vi "matrix-transpose-encapsulate.vi"(11 "output matrix in":T1) -> (3 "output matrix out":T1)   [LabVIEW 2019]
uses:
  <vilib>/Analysis/Matrix/Datatypes/RealMatrix.ctl
  <vilib>/Analysis/Matrix/NI_Matrix.lvlib
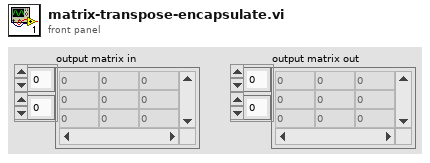
[diagram p1: front panel]
types:
  T1 = typedef "NI_Matrix.lvlib/RealMatrix.ctl" = dbl[][]
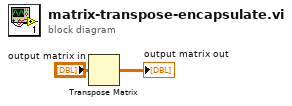
[diagram p0: block diagram]
diagram:
  n1 = Transpose Matrix(1:"output matrix in") -> (0:→"output matrix out":T1)
